vi "FiltroH.vi"(11 "H":dbl) -> (2 "0, 1":u32, 3 "Color":u32(colorbox))   [LabVIEW 2021]
panel:
  in  "Hsup":dbl=230.0 format="%#_13g"
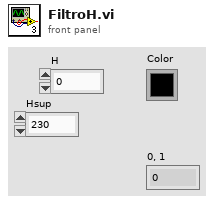
[diagram p1: front panel]
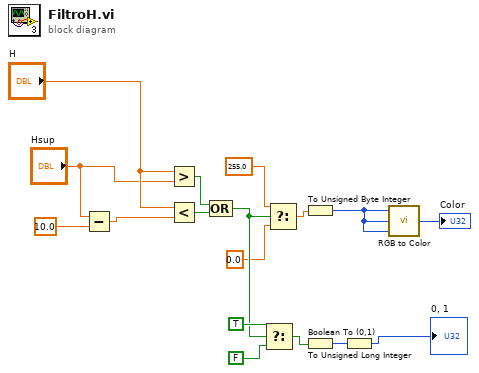
[diagram p0: block diagram]
diagram:
  n1 = Subtract(x="Hsup", y=10.0) -> (x-y=w1:dbl)
  n2 = Greater?(x="H", y="Hsup") -> (0:w4:bool)
  n3 = Less?(x="H", y=w1) -> (x < y?=w5:bool)
  n4 = Compound Arithmetic op=OR(w4, w5) -> (w11:bool)
  n5 = Select(t=TRUE, s=w11, f=FALSE) -> (s? t:f=w14:bool)
  n6 = Select(t=255.0, s=w11, f=0.0) -> (s? t:f=w7:dbl)
  n7 = To Unsigned Byte Integer(number=w7) -> (unsigned 8bit integer=w8:u8)
  n8 = Boolean To (0,1)(Boolean=w14) -> (0, 1=w15:i16)
  n9 = To Unsigned Long Integer(number=w15) -> (unsigned 32bit integer=→"0, 1":u32)
  n10 = call <vilib>:"RGB to Color.vi"("B"=w8, "G"=w8, "R"=w8) -> ("Color"=→"Color":u32)
